vi "Summary header gen.vi"() -> (0 "Header":string)   [LabVIEW 2016]
panel:
  out "array":string[][](array[string])
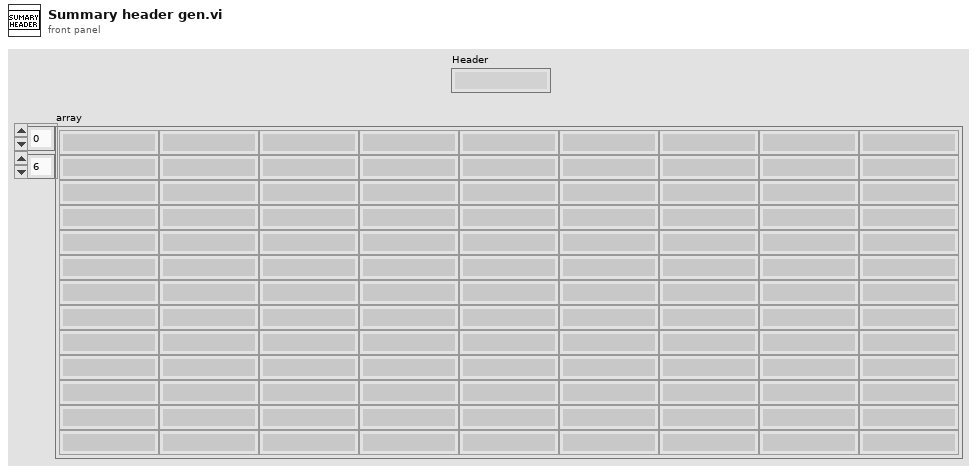
[diagram p1: front panel]
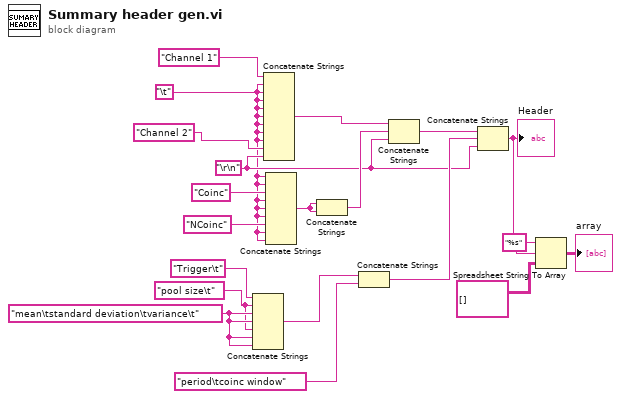
[diagram p0: block diagram]
diagram:
  w10 = "pool size\t"
  w4 = "\r\n"
  w2 = "\t"
  w11 = "mean\tstandard deviation\tvariance\t"
  n1 = Concatenate Strings("Trigger\t", w10, w11, w11, w10, w11, w11) -> (w16:string)
  n2 = Concatenate Strings("Channel 1", w2, w2, w2, w2, w2, w2, w2, w2, "Channel 2", w4) -> (w14:string)
  n3 = Concatenate Strings(w2, w2, "Coinc", w2, w2, w2, "NCoinc", w2, w2) -> (w20:string)
  n4 = Concatenate Strings(w20, w20) -> (w15:string)
  n5 = Concatenate Strings(w16, "period\tcoinc window" ("delimiter (Tab)")) -> (w19:string)
  n6 = Concatenate Strings(w14, w15, w4) -> (w18:string)
  n7 = Concatenate Strings(w18, w19, w4) -> (w7:string)
  "Header" <- w7
  n8 = Spreadsheet String To Array(format string="%s", spreadsheet string=w7, array type (2D Dbl)=string[][] []) -> (array=→"array":string[][])  [unwired: 1 in]
